vi "Initialize Device Core.vi"(8 "error in (no error)":errorcluster, 9 "Reset (F)":bool, 10 "Resource Name":string, 11 "CS++PPG in":refnum<class "CS++PPG.lvclass">) -> (0 "error out":errorcluster, 3 "CS++PPG out":refnum<class "CS++PPG.lvclass">)   [LabVIEW 2016, in "CS++PPG.lvlib" / "CS++PPG.lvclass"]
doc: "Initialize device driver."
uses:
  CS++PPG.lvclass
  CSPP_Core/Actors/CS++DeviceActor/CS++DeviceActor.lvclass
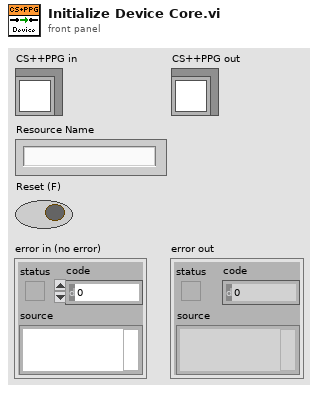
[diagram p1: front panel]
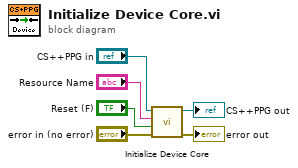
[diagram p0: block diagram]
diagram:
  n1 = call-parent "Initialize Device Core.vi"("error in (no error)"="error in (no error)", "Reset (F)"="Reset (F)", "Resource Name"="Resource Name", "CS++DeviceActor in"="CS++PPG in") -> ("error out"=→"error out":errorcluster, "CS++DeviceActor out"=→"CS++PPG out":refnum<class "CS++PPG.lvclass">)  [unwired: 6 in]
